vi "GetMeas.vi"(1 "VISA resource name":refnum<visa-resource-name>) -> (0 "Numeric Control":dbl)   [LabVIEW 2014]
panel:
  out "element":string
  out "array":string[](array[string])
  out "read buffer":string
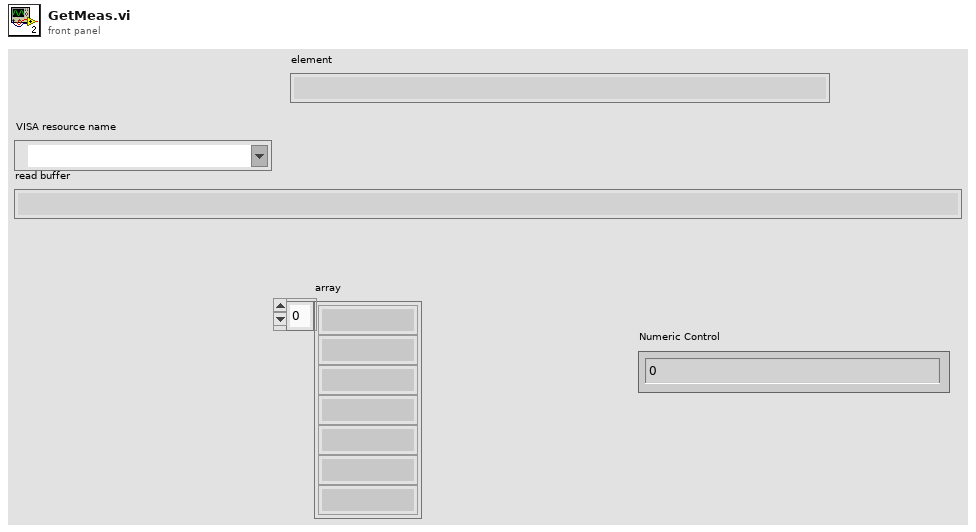
[diagram p1: front panel]
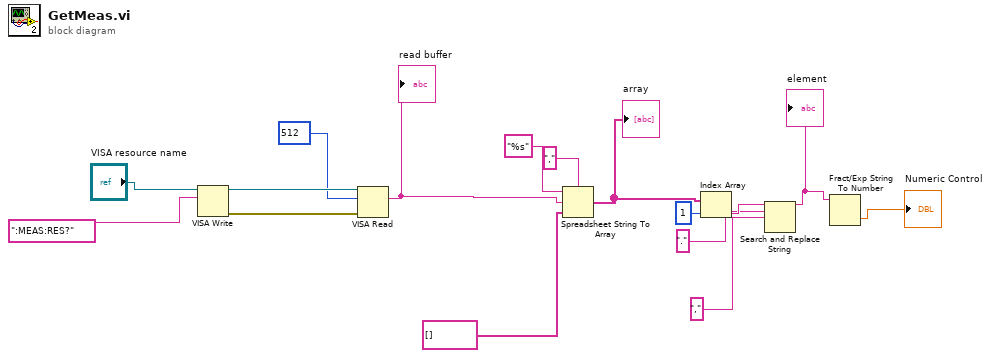
[diagram p0: block diagram]
diagram:
  n1 = VISA Write(VISA resource name="VISA resource name", write buffer=":MEAS:RES?") -> (VISA resource name out=w16:refnum<visa-resource-name>, error out=w15:errorcluster)  [unwired: 1 in, 1 out]
  n2 = VISA Read(VISA resource name=w16, byte count=u32 512, error in (no error)=w15) -> (read buffer=w11:string)  [unwired: 3 out]
  "read buffer" <- w11
  n3 = Spreadsheet String To Array(delimiter (Tab)=",", format string="%s", spreadsheet string=w11, array type (2D Dbl)=string[] []) -> (array=w7:string[])
  "array" <- w7
  n4 = Index Array(array=w7, index=1) -> (element=w4:string)
  n5 = Search and Replace String(input string=w4, search string=".", replace string="," ("replace string (\"\")")) -> (result string=w1:string)  [unwired: 5 in, 3 out]
  "element" <- w1
  n6 = Fract/Exp String To Number(string=w1) -> (number=→"Numeric Control":dbl)  [unwired: 3 in, 1 out]
